vi "GetActualSampleRates.vi"(7 "TimingEngine":T1, 8 "error in":errorcluster, 9 "DAQ Task":refnum<class "DAQ Task.lvclass">, 11 "Chassis Cfg":refnum<class "ChassisCfg.lvclass">) -> (0 "error out":errorcluster, 1 "DAQ Task":refnum<class "DAQ Task.lvclass">, 3 "Chassis Cfg":refnum<class "ChassisCfg.lvclass">)   [LabVIEW 2012, in "Configuration Grandmaster.lvlib" / "ChassisCfg.lvclass"]
uses:
  ChassisCfg.lvclass
  Data Acquisition/Class DAQ Task/DAQ Task.lvclass
  Common/Controls/TE_Designator.ctl
  Data Acquisition/Class DAQ Task/DAQ Task.lvclass/DAQ Task.ctl
  ChassisCfg.lvclass/ChassisCfg.ctl
  Data Acquisition/Class DAQ Task/Read Task.vi
  Data Acquisition/Class DAQ Task/Read All Channels.vi
  Class Timing Group/Write Rate.vi
  Measurements/Class Channel/Channel.lvclass
  <resource>/objmgr/daqmx.rc
  Class Timing Group/TimingGrp.lvclass
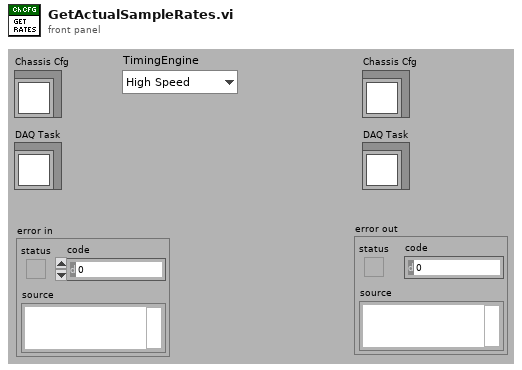
[diagram p1: front panel]
types:
  T1 = typedef "TE_Designator.ctl" = enum16{"High Speed", "Low Speed"}
  T2 = typedef "LS Lock Sizes.ctl" = enum16{"No", "250ms", "500ms", "1s"}
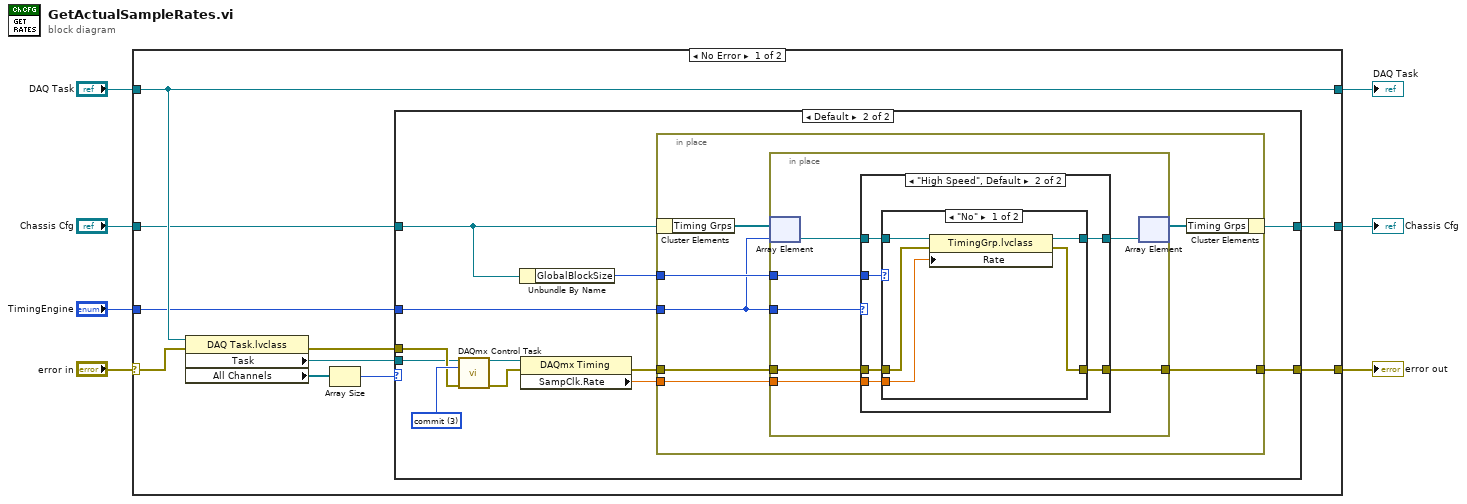
[diagram p0: block diagram]
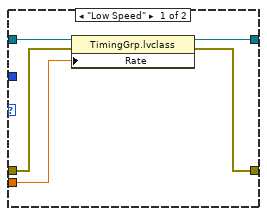
[diagram p3: hidden frame]
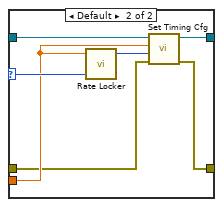
[diagram p4: hidden frame]
diagram:
  n1 = case shown="No Error" "error in" {
    selector: "error in" -> [w15 w69]
    tunnel: [w17 w69] -> w7
    tunnel: "Chassis Cfg" -> [w9 w70]
    tunnel: [w12 w70] -> w5
    tunnel: "DAQ Task" -> [w14 w71]
    tunnel: [w14 w71] -> w2
    tunnel: "TimingEngine" -> [w8 _]
    frame No Error {
      n2 = property class="DAQ Task.lvclass"(reference=w14, error in=w15) -> (error out=w16:errorcluster, "Task"=w13:refnum<k21>, "All Channels"=w11:refnum<class "Channel.lvclass">[])  [unwired: 1 out]
      n3 = Array Size(array=w11) -> (size(s)=w10:i32)
      n4 = case shown="Default" w10 {
        tunnel: [w18 w31] -> w17
        tunnel: w16 -> [w18 w24]
        tunnel: w13 -> [_ w23]
        tunnel: w9 -> [w19 w22]
        tunnel: [w19 w21] -> w12
        tunnel: w8 -> [_ w20]
        frame 0 {
        }
        frame Default {
          w30 = 3 items=["verify"=2, "reserve"=4, "commit"=3, "unreserve"=5, "abort"=6] ("action")
          n5 = call <vilib>:"DAQmx Control Task.vi"("task/channels in"=w23, "action"=w30, "error in"=w24) -> ("task out"=w29:refnum<k21>, "error out"=w28:errorcluster)  [unwired: 11 in]
          n6 = Unbundle By Name(w22) -> ("GlobalBlockSize"=w25:T2)
          n7 = property class="DAQmx Timing"(reference=w29, error in=w28) -> (error out=w26:errorcluster, "SampClk.Rate"=w27:dbl)  [unwired: 1 out]
          n8 = in-place {
            in-place-border: [w38] -> w31
            in-place-border: w27 -> [w37]
            in-place-border: w26 -> [w36]
            in-place-border: w25 -> [w35]
            in-place-border: w20 -> [w33]
            n9 = in-place-cluster #1(w22) -> ("Timing Grps"=w34:refnum<class "TimingGrp.lvclass">[])
            n10 = in-place {
              in-place-border: [w45] -> w38
              in-place-border: w37 -> [w44]
              in-place-border: w36 -> [w43]
              in-place-border: w35 -> [w42]
              in-place-border: w33 -> [w41]
              n11 = in-place-array #2(w34, w33) -> (w40:refnum<class "TimingGrp.lvclass">)
              n12 = case shown="\"High Speed\", Default" w41 {
                tunnel: w44 -> [w46 w56]
                tunnel: w43 -> [w47 w55]
                tunnel: [w48 w54] -> w45
                tunnel: w42 -> [_ w53]
                tunnel: w40 -> [w50 w52]
                tunnel: [w49 w51] -> w39
                frame "Low Speed" {
                  n13 = property class="TimingGrp.lvclass"(reference=w50, error in=w47, "Rate"=w46) -> (reference out=w49:refnum<class "TimingGrp.lvclass">, error out=w48:errorcluster)
                }
                frame "High Speed", Default {
                  n14 = case shown="\"No\"" w53 {
                    selector: w53 -> [_ w68]
                    tunnel: w56 -> [w60 w65]
                    tunnel: w52 -> [w61 w67]
                    tunnel: [w59 w66] -> w51
                    tunnel: w55 -> [w58 w63]
                    tunnel: [w57 w62] -> w54
                    frame "No" {
                      n15 = property class="TimingGrp.lvclass"(reference=w61, error in=w58, "Rate"=w60) -> (reference out=w59:refnum<class "TimingGrp.lvclass">, error out=w57:errorcluster)
                    }
                    frame Default {
                      n16 = call "Rate Locker.vi"("LockToLS"=w68, "HSCfg.Rate"=w65) -> ("HS Block Size"=w64:i32)  [unwired: 1 in, 2 out]
                      n17 = call "Set Timing Cfg.vi"("error in"=w63, "ReadBlk"=w64, "Rate"=w65, "TimingGrp in"=w67) -> ("error out"=w62:errorcluster, "TimingGrp in"=w66:refnum<class "TimingGrp.lvclass">)  [unwired: 6 in]
                    }
                  }
                }
              }
              n18 = in-place-array #2(w39) -> (w32:refnum<class "TimingGrp.lvclass">[])  [unwired: 1 out]
            }
            n19 = in-place-cluster #1("Timing Grps"=w32) -> (w21:refnum<class "ChassisCfg.lvclass">)
          }
        }
      }
    }
    frame Error {
    }
  }
  "error out" <- w7
  "Chassis Cfg" <- w5
  "DAQ Task" <- w2
